vi "Matrix_ExtractRowVector.vi"(10 "Row":i32, 11 "input matrix":T1) -> (0 "Error":bool, 3 "output row":T1)   [LabVIEW 2019, in "Trajectory_Library.lvlib"]
doc: "Extracts a given row into a row vector with new underlying storage.\n \nInputs:\n - input matrix -- The input matrix\n - row -- The row to extract a vector from.\n\nOutputs:\n - output row -- A row vector from the given row.\n - error -- If TRUE, an error occured."
uses:
  Trajectory_Library.lvlib
  <vilib>/Analysis/Matrix/Datatypes/RealMatrix.ctl
  <vilib>/Analysis/Matrix/NI_Matrix.lvlib
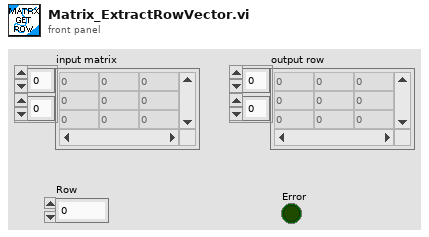
[diagram p1: front panel]
types:
  T1 = typedef "NI_Matrix.lvlib/RealMatrix.ctl" = dbl[][]
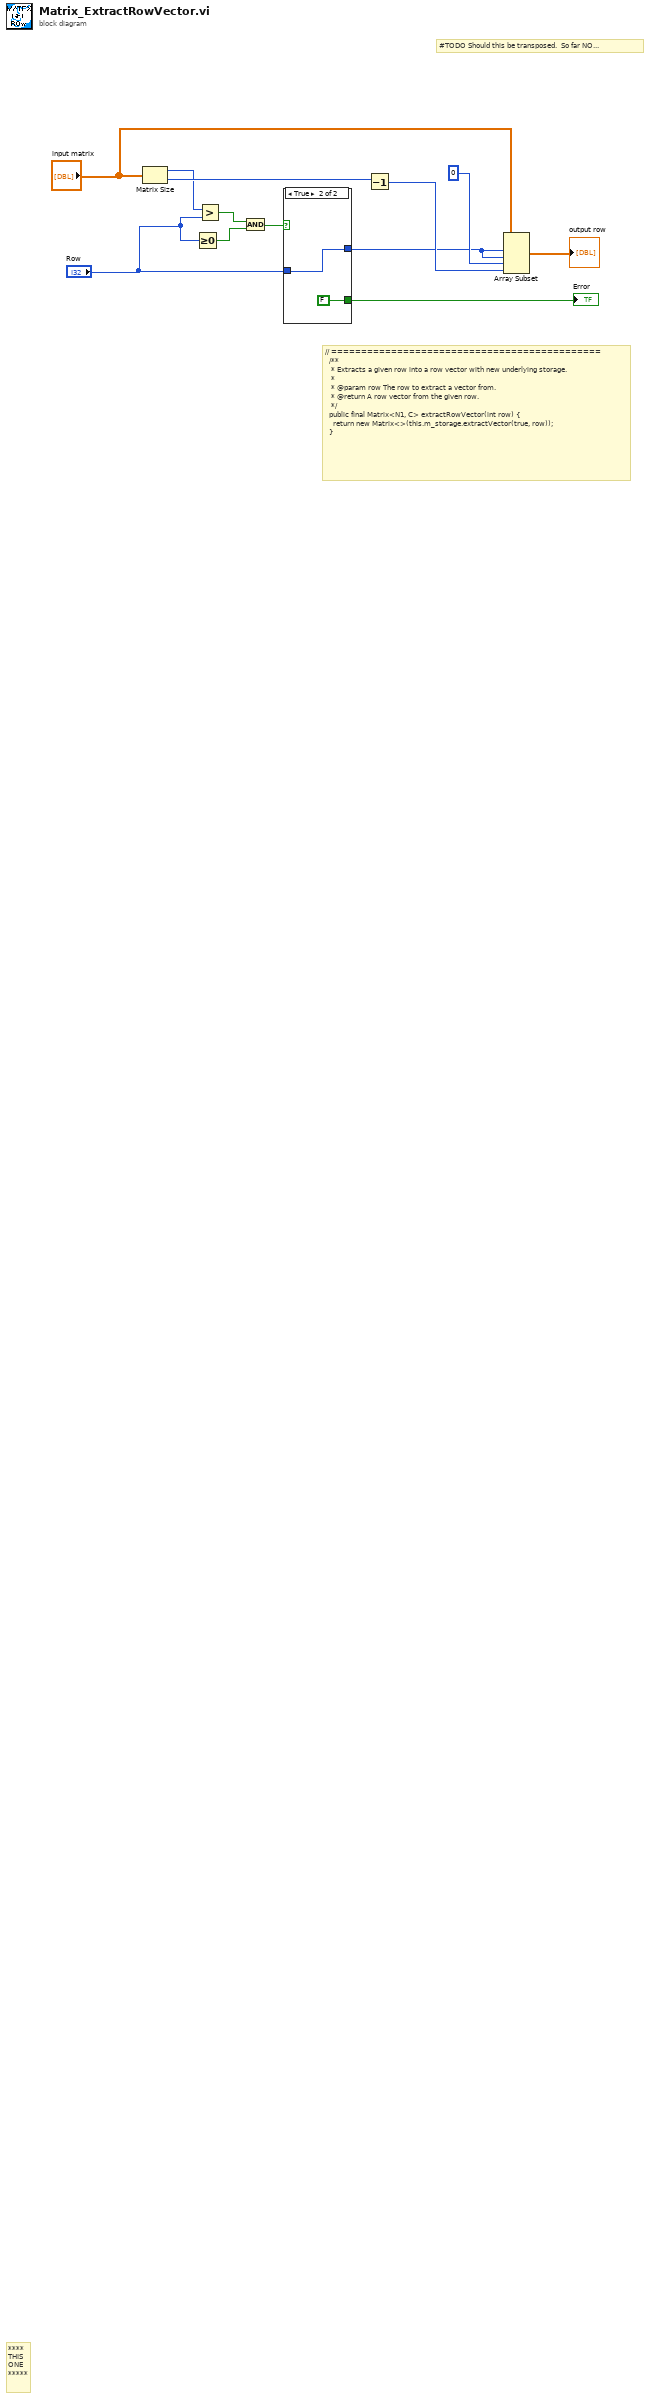
[diagram p0: block diagram]
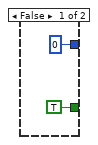
[diagram p2: hidden frame]
diagram:
  # "#TODO Should this be transposed.  So far NO..."
  # "// =============================================\n  /**\n   * Extracts a given row into a row vector with new underlying storage.\n   *\n   * @param row The row to extract a vector from.\n   * @return A row vector from the given row.\n   */\n  public final Matrix<N1, C> extractRowVector(int row) {\n    return new Matrix<>(this.m_storage.extractVector(true, row));\n  }"
  # "****\nTHIS\nONE\n*****"
  n1 = Matrix Size(0:"input matrix") -> (1:w7:i32, 2:w10:i32)
  n2 = Greater Or Equal To 0?(x="Row") -> (x >= 0?=w8:bool)
  n3 = Greater?(x=w7, y="Row") -> (0:w9:bool)
  n4 = And(x=w9, y=w8) -> (x .and. y?=w4:bool)
  n5 = case shown="True" w4 {
    tunnel: "Row" -> [_ w16]
    tunnel: [0 ("Row") w16] -> w2
    tunnel: [TRUE FALSE] -> w1
    frame False {
    }
    frame True {
    }
  }
  "Error" <- w1
  n6 = Decrement(x=w10) -> (x-1=w5:i32)
  n7 = Array Subset(array="input matrix", index (row)=w2, length (row)=w2, index (col)=0 ("row 1"), length (col)=w5) -> (→"output row":T1)
